vi "grSim Packet Command UDP Test.vi"(4 "FIRASim?":bool=TRUE, 6 "grSim replacement":T3={"grSim_RobotReplacement"=[{"x"=0.0, "y"=-450.0, "dir"=0.0, "yellowteam"=FALSE, "id"=0}, {"x"=0.0, "y"=-270.0, "dir"=0.0, "yellowteam"=FALSE, "id"=1}, {"x"=0.0, "y"=-90.0, "dir"=0.0, "yellowteam"=FALSE, "id"=2}, {"x"=0.0, "y"=90.0, "dir"=0.0, "yellowteam"=FALSE, "id"=3}, {"x"=0.0, "y"=270.0, "dir"=0.0, "yellowteam"=FALSE, "id"=4}, {"x"=0.0, "y"=450.0, "dir"=0.0, "yellowteam"=FALSE, "id"=5}], "grSim_BallReplacement"={"x"=0.0, "y"=0.0, "vx"=0.0, "vy"=0.0}}, 7 "replace ball":bool, 8 "Port:":u16=20011, 9 "SSL Vision Address:":string="127.0.0.1", 10 "isteamyellow":bool=TRUE, 11 "Robots":T4[](array[typedef])) -> ()   [LabVIEW 2023]
uses:
  Convert AI Robot to Robot Command Folder/grSim/grSim Robot Command.ctl
  grSim RobotReplacement.ctl
  grSim_BallReplacement.ctl
panel:
  out "error out":errorcluster
  out "Array":u8[](array[numeric]) format="%02x"
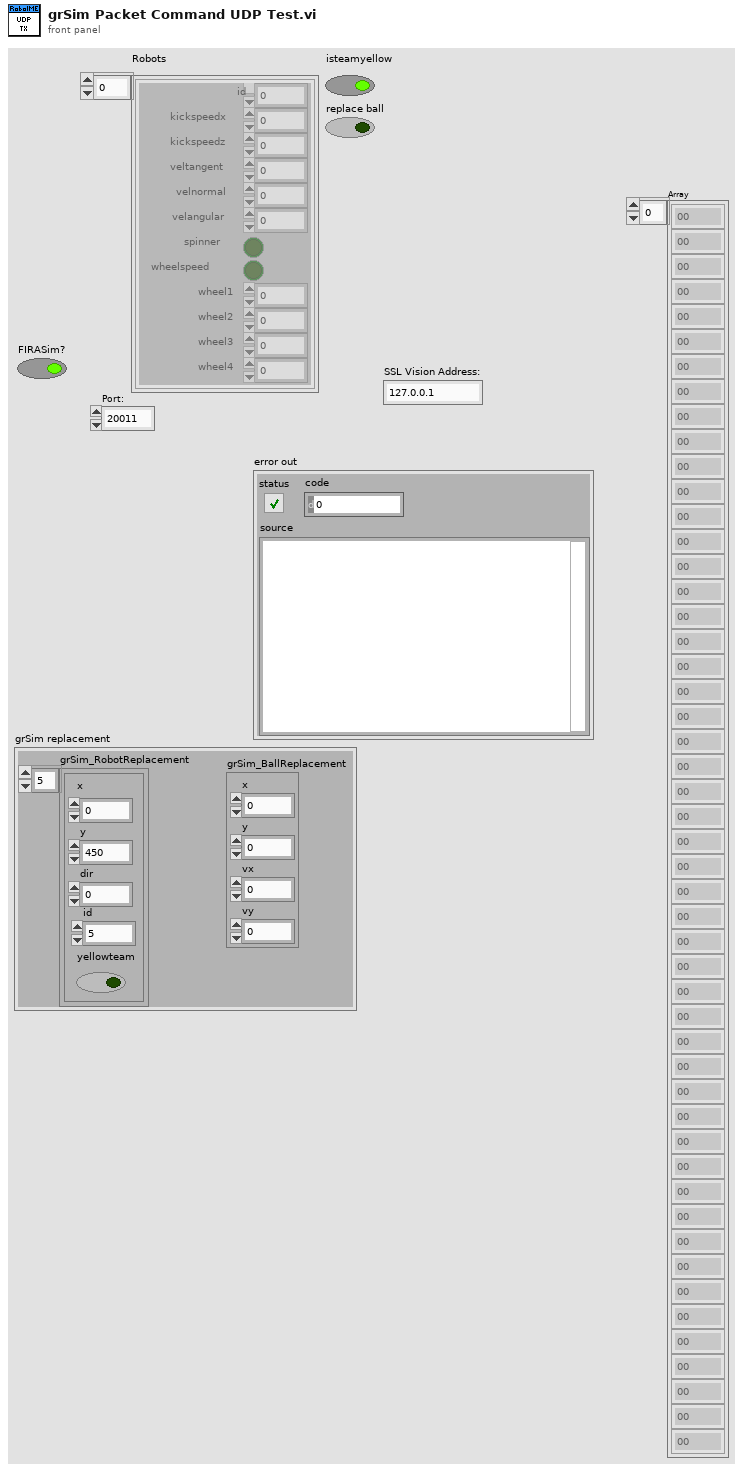
[diagram p1: front panel]
types:
  T1 = typedef "grSim RobotReplacement.ctl" = cluster{"x":dbl, "y":dbl, "dir":dbl, "yellowteam":bool, "id":u32}
  T2 = typedef "grSim_BallReplacement.ctl" = cluster{"x":dbl, "y":dbl, "vx":dbl, "vy":dbl}
  T3 = cluster{"grSim_RobotReplacement":T1[], "grSim_BallReplacement":T2}
  T4 = typedef "grSim Robot Command.ctl" = cluster{"id":u32, "kickspeedx":sgl, "kickspeedz":sgl, "veltangent":sgl, "velnormal":sgl, "velangular":sgl, "spinner":bool, "wheelspeed":bool, "wheel1":sgl, "wheel2":sgl, "wheel3":sgl, "wheel4":sgl}
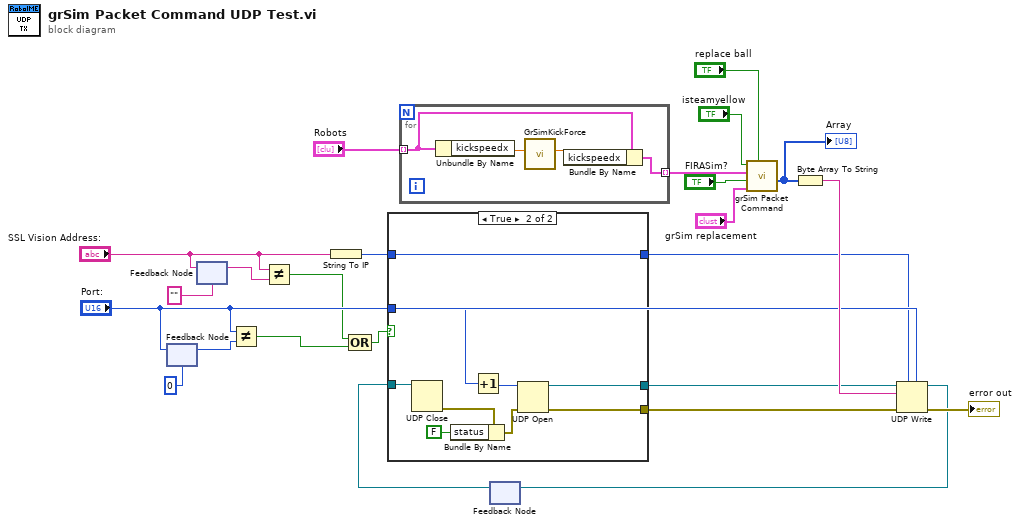
[diagram p0: block diagram]
diagram:
  n1 = feedback #1(u16 0 ("Port:")) -> (w21:u16)
  n2 = feedback-in #1("Port:") -> ()
  n3 = feedback #2("" ("SSL Vision Address:")) -> (w19:string)
  n4 = feedback-in #2("SSL Vision Address:") -> ()
  n5 = Not Equal?(x="Port:", y=w21) -> (x != y?=w17:bool)
  n6 = Not Equal?(x="SSL Vision Address:", y=w19) -> (x != y?=w18:bool)
  n7 = String To IP(1:"SSL Vision Address:") -> (0:w8:u32)
  n8 = Compound Arithmetic op=OR(w18, w17) -> (w16:bool)
  n9 = for {
    tunnel: "Robots" -> [w28] mode=indexing
    tunnel: [w27] -> w5 mode=indexing
    n10 = Unbundle By Name(w28) -> ("kickspeedx"=w26:sgl)
    n11 = call "GrSimKickForce.vi"("real kick"=w26) -> ("grsim kick"=w25:dbl)  [unwired: 10 in]
    n12 = Bundle By Name(cluster=w28, "kickspeedx"=w25) -> (w27:T4)
  }
  n13 = feedback #3() -> (w14:refnum<k16>)  [unwired: 1 in]
  n14 = case shown="True" w16 {
    tunnel: [_ w39] -> w22
    tunnel: [w30 w37] -> w13
    tunnel: "Port:" -> [_ w36]
    tunnel: w8 -> [w29 w34]
    tunnel: w14 -> [w30 w35]
    tunnel: [w29 w34] -> w7
    frame False {
    }
    frame True {
      n15 = UDP Close(connection ID=w35) -> (error out=w33:errorcluster)  [unwired: 1 in, 1 out]
      n16 = Bundle By Name(cluster=w33, "status"=FALSE) -> (w32:errorcluster)
      n17 = Increment(x=w36) -> (x+1=w38:u16)
      n18 = UDP Open(8:w32, 11:w38) -> (port=w37:refnum<k16>, 0:w39:errorcluster)  [unwired: 3 in, 1 out]
    }
  }
  n19 = call "grSim Packet Command.vi"("replace ball"="replace ball", "grSim replacement"="grSim replacement", "FIRASim?"="FIRASim?", "Robots"=w5, "isteamyellow"="isteamyellow") -> ("Array"=w4:u8[])  [unwired: 6 in]
  "Array" <- w4
  n20 = Byte Array To String(unsigned byte array=w4) -> (string=w23:string)
  n21 = UDP Write(address=w7, port or service name="Port:", connection ID=w13, data in=w23, 8:w22) -> (error out=→"error out":errorcluster, 3:w12:refnum<k16>)  [unwired: 1 in]
  n22 = feedback-in #3(w12) -> ()
